vi "nanocal -- nuclear schottky fit V8.vi"() -> ()   [LabVIEW 2021] (continued)
\"τ22\" -> 0.000000000000   ,  \"τN1\" -> 0.000000000000   ,  \"τN2\" -> 0.000000000000   ,  \"σηlogτ1 \" -> 0.000000000000   ,  \"σηlogτS\" -> 0.000000000000   ,  \"σηlogτN\" -> 0.000000000000   ,  \"σlogτ1\" -> 0.000000000000   ,  \"σlogτS\" -> 0.000000000000   ,  \"σlogτN\" -> 0.000000000000   ,  \"σητ1\" -> 0.000000000000   ,  \"σητS \" -> 0.000000000000   ,  \"σητN\" -> 0.000000000000    |>   , \r\"IDS0361_210908_RAW_cal__ref_\" ->   <|    \"ζ\" -> 0.274843315726   ,  \"τ1\" -> 0.065669556126   ,  \"τS\" -> 0.043737045326   ,  \"τN\" -> 0.171424826572   ,  \"τC\" -> 0.000899266573   ,  \"κ0\" -> 0.000000000755   ,  \"mm1\" -> 0.000191414578   ,  \"mm2\" -> 0.011258128300   ,  \"mm3\" -> 0.329416954010   ,  \"T\" -> 0.168000000000   ,  \"B\" -> 12.000000000000   ,  \"θ\" -> 60.000000000000   ,  \"Reoff\" -> 0.000000000000   ,  \"Imoff\" -> 0.000000000000   ,  \"στ1\" -> 0.000077610156   ,  \"στS\" -> 0.000022738638   ,  \"στN\" -> 0.000144137782   ,  \"τ11 \" -> 0.000000000000   ,  \"τ12\" -> 0.000000000000   ,  \"τ22\" -> 0.000000000000   ,  \"τN1\" -> 0.000000000000   ,  \"τN2\" -> 0.000000000000   ,  \"σηlogτ1 \" -> 0.041134517971   ,  \"σηlogτS\" -> 0.001768570492   ,  \"σηlogτN\" -> 0.052373530031   ,  \"σlogτ1\" -> 0.001181828544   ,  \"σlogτS\" -> 0.000519894231   ,  \"σlogτN\" -> 0.000840822097   ,  \"σητ1\" -> 0.002701285537   ,  \"σητS \" -> 0.000077352048   ,  \"σητN\" -> 0.008978123302    |>   , \r\"IDS0361_210908_RAW_cal__sam_\" ->   <|    \"ζ\" -> 0.166104690940   ,  \"τ1\" -> 0.071049175548   ,  \"τS\" -> 0.068661809155   ,  \"τN\" -> 0.222482953546   ,  \"τC\" -> 0.001364223445   ,  \"κ0\" -> 0.000000000861   ,  \"mm1\" -> 0.000191495940   ,  \"mm2\" -> 0.014533832786   ,  \"mm3\" -> 0.397193343795   ,  \"T\" -> 0.168000000000   ,  \"B\" -> 12.000000000000   ,  \"θ\" -> 60.000000000000   ,  \"Reoff\" -> -34789156.626506023100   ,  \"Imoff\" -> 0.000000000000   ,  \"στ1\" -> 0.000000000000   ,  \"στS\" -> 0.000000000000   ,  \"στN\" -> 0.000000000000   ,  \"τ11 \" -> 0.000000000000   ,  \"τ12\" -> 0.000000000000   ,  \"τ22\" -> 0.000000000000   ,  \"τN1\" -> 0.000000000000   ,  \"τN2\" -> 0.000000000000   ,  \"σηlogτ1 \" -> 0.000000000000   ,  \"σηlogτS\" -> 0.000000000000   ,  \"σηlogτN\" -> 0.000000000000   ,  \"σlogτ1\" -> 0.000000000000   ,  \"σlogτS\" -> 0.000000000000   ,  \"σlogτN\" -> 0.000000000000   ,  \"σητ1\" -> 0.000000000000   ,  \"σητS \" -> 0.000000000000   ,  \"σητN\" -> 0.000000000000    |>   , \r\"IDS0362_210908_RAW_cal__ref_\" ->   <|    \"ζ\" -> 0.210826162252   ,  \"τ1\" -> 0.054763021259   ,  \"τS\" -> 0.037603010957   ,  \"τN\" -> 0.089871422671   ,  \"τC\" -> 0.000959483183   ,  \"κ0\" -> 0.000000001045   ,  \"mm1\" -> 0.000164174443   ,  \"mm2\" -> 0.012877562256   ,  \"mm3\" -> 0.197030146997   ,  \"T\" -> 0.197000000000   ,  \"B\" -> 12.000000000000   ,  \"θ\" -> 60.000000000000   ,  \"Reoff\" -> 0.000000000000   ,  \"Imoff\" -> 0.000000000000   ,  \"στ1\" -> 0.000049220168   ,  \"στS\" -> 0.000011686979   ,  \"στN\" -> 0.000056446769   ,  \"τ11 \" -> 0.000000000000   ,  \"τ12\" -> 0.000000000000   ,  \"τ22\" -> 0.000000000000   ,  \"τN1\" -> 0.000000000000   ,  \"τN2\" -> 0.000000000000   ,  \"σηlogτ1 \" -> 0.038148915938   ,  \"σηlogτS\" -> 0.001374810052   ,  \"σηlogτN\" -> 0.048522876787   ,  \"σlogτ1\" -> 0.000898784750   ,  \"σlogτS\" -> 0.000310799031   ,  \"σlogτN\" -> 0.000628083622   ,  \"σητ1\" -> 0.002089149895   ,  \"σητS \" -> 0.000051696997   ,  \"σητN\" -> 0.004360819969    |>   , \r\"IDS0362_210908_RAW_cal__sam_\" ->   <|    \"ζ\" -> 0.123741217510   ,  \"τ1\" -> 0.059103977068   ,  \"τS\" -> 0.051096152058   ,  \"τN\" -> 0.122661863704   ,  \"τC\" -> 0.001502836172   ,  \"κ0\" -> 0.000000001149   ,  \"mm1\" -> 0.000161683871   ,  \"mm2\" -> 0.014394250129   ,  \"mm3\" -> 0.241309923424   ,  \"T\" -> 0.197000000000   ,  \"B\" -> 12.000000000000   ,  \"θ\" -> 60.000000000000   ,  \"Reoff\" -> -17448795.180722892300   ,  \"Imoff\" -> 0.000000000000   ,  \"στ1\" -> 0.000000000000   ,  \"στS\" -> 0.000000000000   ,  \"στN\" -> 0.000000000000   ,  \"τ11 \" -> 0.000000000000   ,  \"τ12\" -> 0.000000000000   ,  \"τ22\" -> 0.000000000000   ,  \"τN1\" -> 0.000000000000   ,  \"τN2\" -> 0.000000000000   ,  \"σηlogτ1 \" -> 0.000000000000   ,  \"σηlogτS\" -> 0.000000000000   ,  \"σηlogτN\" -> 0.000000000000   ,  \"σlogτ1\" -> 0.000000000000   ,  \"σlogτS\" -> 0.000000000000   ,  \"σlogτN\" -> 0.000000000000   ,  \"σητ1\" -> 0.000000000000   ,  \"σητS \" -> 0.000000000000   ,  \"σητN\" -> 0.000000000000    |>   , \r\"IDS0363_210908_RAW_cal__ref_\" ->   <|    \"ζ\" -> 0.120195011159   ,  \"τ1\" -> 0.037982415348   ,  \"τS\" -> 0.029921195592   ,  \"τN\" -> 0.032714371407   ,  \"τC\" -> 0.001103711032   ,  \"κ0\" -> 0.000000001361   ,  \"mm1\" -> 0.000115022123   ,  \"mm2\" -> 0.013740329759   ,  \"mm3\" -> 0.095394824172   ,  \"T\" -> 0.250000000000   ,  \"B\" -> 12.000000000000   ,  \"θ\" -> 60.000000000000   ,  \"Reoff\" -> 0.000000000000   ,  \"Imoff\" -> 0.000000000000   ,  \"στ1\" -> 0.000012313434   ,  \"στS\" -> 0.000002128775   ,  \"στN\" -> 0.000006964176   ,  \"τ11 \" -> 0.000000000000   ,  \"τ12\" -> 0.000000000000   ,  \"τ22\" -> 0.000000000000   ,  \"τN1\" -> 0.000000000000   ,  \"τN2\" -> 0.000000000000   ,  \"σηlogτ1 \" -> 0.037050900153   ,  \"σηlogτS\" -> 0.000901906922   ,  \"σηlogτN\" -> 0.045689519095   ,  \"σlogτ1\" -> 0.000324187744   ,  \"σlogτS\" -> 0.000071146055   ,  \"σlogτN\" -> 0.000212878182   ,  \"σητ1\" -> 0.001407282679   ,  \"σητS \" -> 0.000026986133   ,  \"σητN\" -> 0.001494703897    |>   , \r\"IDS0363_210908_RAW_cal__sam_\" ->   <|    \"ζ\" -> 0.074359211271   ,  \"τ1\" -> 0.044477620306   ,  \"τS\" -> 0.040449563551   ,  \"τN\" -> 0.044745540249   ,  \"τC\" -> 0.001712765821   ,  \"κ0\" -> 0.000000001493   ,  \"mm1\" -> 0.000114327803   ,  \"mm2\" -> 0.016556677808   ,  \"mm3\" -> 0.121049525039   ,  \"T\" -> 0.250000000000   ,  \"B\" -> 12.000000000000   ,  \"θ\" -> 60.000000000000   ,  \"Reoff\" -> -10147590.361445784600   ,  \"Imoff\" -> 0.000000000000   ,  \"στ1\" -> 0.000000000000   ,  \"στS\" -> 0.000000000000   ,  \"στN\" -> 0.000000000000   ,  \"τ11 \" -> 0.000000000000   ,  \"τ12\" -> 0.000000000000   ,  \"τ22\" -> 0.000000000000   ,  \"τN1\" -> 0.000000000000   ,  \"τN2\" -> 0.000000000000   ,  \"σηlogτ1 \" -> 0.000000000000   ,  \"σηlogτS\" -> 0.000000000000   ,  \"σηlogτN\" -> 0.000000000000   ,  \"σlogτ1\" -> 0.000000000000   ,  \"σlogτS\" -> 0.000000000000   ,  \"σlogτN\" -> 0.000000000000   ,  \"σητ1\" -> 0.000000000000   ,  \"σητS \" -> 0.000000000000   ,  \"σητN\" -> 0.000000000000    |>   , \r\"IDS0364_210908_RAW_cal__ref_\" ->   <|    \"ζ\" -> 0.081935948170   ,  \"τ1\" -> 0.032287614632   ,  \"τS\" -> 0.026949270434   ,  \"τN\" -> 0.016861876648   ,  \"τC\" -> 0.001338410345   ,  \"κ0\" -> 0.000000001744   ,  \"mm1\" -> 0.000097212898   ,  \"mm2\" -> 0.014855671361   ,  \"mm3\" -> 0.066073995677   ,  \"T\" -> 0.307000000000   ,  \"B\" -> 12.000000000000   ,  \"θ\" -> 60.000000000000   ,  \"Reoff\" -> 0.000000000000   ,  \"Imoff\" -> 0.000000000000   ,  \"στ1\" -> 0.000017118957   ,  \"στS\" -> 0.000002077535   ,  \"στN\" -> 0.000005632909   ,  \"τ11 \" -> 0.000000000000   ,  \"τ12\" -> 0.000000000000   ,  \"τ22\" -> 0.000000000000   ,  \"τN1\" -> 0.000000000000   ,  \"τN2\" -> 0.000000000000   ,  \"σηlogτ1 \" -> 0.036879495168   ,  \"σηlogτS\" -> 0.000607281388   ,  \"σηlogτN\" -> 0.044616936261   ,  \"σlogτ1\" -> 0.000530201983   ,  \"σlogτS\" -> 0.000077090575   ,  \"σlogτN\" -> 0.000334061782   ,  \"σητ1\" -> 0.001190750928   ,  \"σητS \" -> 0.000016365790   ,  \"σητN\" -> 0.000752325276    |>   , \r\"IDS0364_210908_RAW_cal__sam_\" ->   <|    \"ζ\" -> 0.051560123380   ,  \"τ1\" -> 0.037167172913   ,  \"τS\" -> 0.035875072163   ,  \"τN\" -> 0.021782945969   ,  \"τC\" -> 0.002191662682   ,  \"κ0\" -> 0.000000001902   ,  \"mm1\" -> 0.000101812126   ,  \"mm2\" -> 0.018093196790   ,  \"mm3\" -> 0.081794699340   ,  \"T\" -> 0.307000000000   ,  \"B\" -> 12.000000000000   ,  \"θ\" -> 60.000000000000   ,  \"Reoff\" -> -5584337.349397592250   ,  \"Imoff\" -> 0.000000000000   ,  \"στ1\" -> 0.000000000000   ,  \"στS\" -> 0.000000000000   ,  \"στN\" -> 0.000000000000   ,  \"τ11 \" -> 0.000000000000   ,  \"τ12\" -> 0.000000000000   ,  \"τ22\" -> 0.000000000000   ,  \"τN1\" -> 0.000000000000   ,  \"τN2\" -> 0.000000000000   ,  \"σηlogτ1 \" -> 0.000000000000   ,  \"σηlogτS\" -> 0.000000000000   ,  \"σηlogτN\" -> 0.000000000000   ,  \"σlogτ1\" -> 0.000000000000   ,  \"σlogτS\" -> 0.000000000000   ,  \"σlogτN\" -> 0.000000000000   ,  \"σητ1\" -> 0.000000000000   ,  \"σητS \" -> 0.000000000000   ,  \"σητN\" -> 0.000000000000    |>   , \r\"IDS0365_210908_RAW_cal__ref_\" ->   <|    \"ζ\" -> 0.060609447021   ,  \"τ1\" -> 0.026924433713   ,  \"τS\" -> 0.025092686079   ,  \"τN\" -> 0.009588284117   ,  \"τC\" -> 0.001648006453   ,  \"κ0\" -> 0.000000002119   ,  \"mm1\" -> 0.000088958851   ,  \"mm2\" -> 0.015130564959   ,  \"mm3\" -> 0.050135880977   ,  \"T\" -> 0.360000000000   ,  \"B\" -> 12.000000000000   ,  \"θ\" -> 60.000000000000   ,  \"Reoff\" -> 0.000000000000   ,  \"Imoff\" -> 0.000000000000   ,  \"στ1\" -> 0.000013873165   ,  \"στS\" -> 0.000001316641   ,  \"στN\" -> 0.000002948025   ,  \"τ11 \" -> 0.000000000000   ,  \"τ12\" -> 0.000000000000   ,  \"τ22\" -> 0.000000000000   ,  \"τN1\" -> 0.000000000000   ,  \"τN2\" -> 0.000000000000   ,  \"σηlogτ1 \" -> 0.038447991520   ,  \"σηlogτS\" -> 0.000466260948   ,  \"σηlogτN\" -> 0.044499975786   ,  \"σlogτ1\" -> 0.000515263014   ,  \"σlogτS\" -> 0.000052471110   ,  \"σlogτN\" -> 0.000307461145   ,  \"σητ1\" -> 0.001035190399   ,  \"σητS \" -> 0.000011699740   ,  \"σητN\" -> 0.000426678411    |>   , \r\"IDS0365_210908_RAW_cal__sam_\" ->   <|    \"ζ\" -> 0.037527154631   ,  \"τ1\" -> 0.031791574880   ,  \"τS\" -> 0.032568278603   ,  \"τN\" -> 0.012463984296   ,  \"τC\" -> 0.002682405917   ,  \"κ0\" -> 0.000000002306   ,  \"mm1\" -> 0.000090102201   ,  \"mm2\" -> 0.018466994147   ,  \"mm3\" -> 0.062639080041   ,  \"T\" -> 0.360000000000   ,  \"B\" -> 12.000000000000   ,  \"θ\" -> 60.000000000000   ,  \"Reoff\" -> -2846385.542168676850   ,  \"Imoff\" -> 0.000000000000   ,  \"στ1\" -> 0.000000000000   ,  \"στS\" -> 0.000000000000   ,  \"στN\" -> 0.000000000000   ,  \"τ11 \" -> 0.000000000000   ,  \"τ12\" -> 0.000000000000   ,  \"τ22\" -> 0.000000000000   ,  \"τN1\" -> 0.000000000000   ,  \"τN2\" -> 0.000000000000   ,  \"σηlogτ1 \" -> 0.000000000000   ,  \"σηlogτS\" -> 0.000000000000   ,  \"σηlogτN\" -> 0.000000000000   ,  \"σlogτ1\" -> 0.000000000000   ,  \"σlogτS\" -> 0.000000000000   ,  \"σlogτN\" -> 0.000000000000   ,  \"σητ1\" -> 0.000000000000   ,  \"σητS \" -> 0.000000000000   ,  \"σητN\" -> 0.000000000000    |>   , \r\"IDS0366_210908_RAW_cal__ref_\" ->   <|    \"ζ\" -> 0.044599134979   ,  \"τ1\" -> 0.022455429279   ,  \"τS\" -> 0.023337915843   ,  \"τN\" -> 0.005128755710   ,  \"τC\" -> 0.001792889841   ,  \"κ0\" -> 0.000000002649   ,  \"mm1\" -> 0.000071495516   ,  \"mm2\" -> 0.015101682830   ,  \"mm3\" -> 0.038811401254   ,  \"T\" -> 0.430000000000   ,  \"B\" -> 12.000000000000   ,  \"θ\" -> 60.000000000000   ,  \"Reoff\" -> 0.000000000000   ,  \"Imoff\" -> 0.000000000000   ,  \"στ1\" -> 0.000015607545   ,  \"στS\" -> 0.000001063228   ,  \"στN\" -> 0.000002022209   ,  \"τ11 \" -> 0.000000000000   ,  \"τ12\" -> 0.000000000000   ,  \"τ22\" -> 0.000000000000   ,  \"τN1\" -> 0.000000000000   ,  \"τN2\" -> 0.000000000000   ,  \"σηlogτ1 \" -> 0.040328561350   ,  \"σηlogτS\" -> 0.000330725156   ,  \"σηlogτN\" -> 0.044548205014   ,  \"σlogτ1\" -> 0.000695045482   ,  \"σlogτS\" -> 0.000045557962   ,  \"σlogτN\" -> 0.000394288447   ,  \"σητ1\" -> 0.000905595157   ,  \"σητS \" -> 0.000007718436   ,  \"σητN\" -> 0.000228476861    |>   , \r\"IDS0366_210908_RAW_cal__sam_\" ->   <|    \"ζ\" -> 0.029143715364   ,  \"τ1\" -> 0.026198855926   ,  \"τS\" -> 0.029745373312   ,  \"τN\" -> 0.006649011545   ,  \"τC\" -> 0.003090491846   ,  \"κ0\" -> 0.000000002869   ,  \"mm1\" -> 0.000079676072   ,  \"mm2\" -> 0.018163106475   ,  \"mm3\" -> 0.048501617675   ,  \"T\" -> 0.430000000000   ,  \"B\" -> 12.000000000000   ,  \"θ\" -> 60.000000000000   ,  \"Reoff\" -> -2237951.807228915390   ,  \"Imoff\" -> 0.000000000000   ,  \"στ1\" -> 0.000000000000   ,  \"στS\" -> 0.000000000000   ,  \"στN\" -> 0.000000000000   ,  \"τ11 \" -> 0.000000000000   ,  \"τ12\" -> 0.000000000000   ,  \"τ22\" -> 0.000000000000   ,  \"τN1\" -> 0.000000000000   ,  \"τN2\" -> 0.000000000000   ,  \"σηlogτ1 \" -> 0.000000000000   ,  \"σηlogτS\" -> 0.000000000000   ,  \"σηlogτN\" -> 0.000000000000   ,  \"σlogτ1\" -> 0.000000000000   ,  \"σlogτS\" -> 0.000000000000   ,  \"σlogτN\" -> 0.000000000000   ,  \"σητ1\" -> 0.000000000000   ,  \"σητS \" -> 0.000000000000   ,  \"σητN\" -> 0.000000000000    |>   , \r\"IDS0367_210908_RAW_cal__ref_\" ->   <|    \"ζ\" -> 0.034740009221   ,  \"τ1\" -> 0.017028751834   ,  \"τS\" -> 0.022162435410   ,  \"τN\" -> 0.002809238258   ,  \"τC\" -> 0.001913219314   ,  \"κ0\" -> 0.000000003308   ,  \"mm1\" -> 0.000059427665   ,  \"mm2\" -> 0.013533798262   ,  \"mm3\" -> 0.031187935063   ,  \"T\" -> 0.530000000000   ,  \"B\" -> 12.000000000000   ,  \"θ\" -> 60.000000000000   ,  \"Reoff\" -> 0.000000000000   ,  \"Imoff\" -> 0.000000000000   ,  \"στ1\" -> 0.000027033003   ,  \"στS\" -> 0.000001554115   ,  \"στN\" -> 0.000002352999   ,  \"τ11 \" -> 0.000000000000   ,  \"τ12\" -> 0.000000000000   ,  \"τ22\" -> 0.000000000000   ,  \"τN1\" -> 0.000000000000   ,  \"τN2\" -> 0.000000000000   ,  \"σηlogτ1 \" -> 0.045416924257   ,  \"σηlogτS\" -> 0.000278228215   ,  \"σηlogτN\" -> 0.045395504019   ,  \"σlogτ1\" -> 0.001587491763   ,  \"σlogτS\" -> 0.000070123814   ,  \"σlogτN\" -> 0.000837593181   ,  \"σητ1\" -> 0.000773393532   ,  \"σητS \" -> 0.000006166215   ,  \"σητN\" -> 0.000127526787    |>   , \r\"IDS0367_210908_RAW_cal__sam_\" ->   <|    \"ζ\" -> 0.024637271207   ,  \"τ1\" -> 0.025634847148   ,  \"τS\" -> 0.027302474030   ,  \"τN\" -> 0.003538185279   ,  \"τC\" -> 0.003933377133   ,  \"κ0\" -> 0.000000003566   ,  \"mm1\" -> 0.000083131278   ,  \"mm2\" -> 0.019726981228   ,  \"mm3\" -> 0.041358600771   ,  \"T\" -> 0.530000000000   ,  \"B\" -> 12.000000000000   ,  \"θ\" -> 60.000000000000   ,  \"Reoff\" -> -1629518.072289161380   ,  \"Imoff\" -> 0.000000000000   ,  \"στ1\" -> 0.000000000000   ,  \"στS\" -> 0.000000000000   ,  \"στN\" -> 0.000000000000   ,  \"τ11 \" -> 0.000000000000   ,  \"τ12\" -> 0.000000000000   ,  \"τ22\" -> 0.000000000000   ,  \"τN1\" -> 0.000000000000   ,  \"τN2\" -> 0.000000000000   ,  \"σηlogτ1 \" -> 0.000000000000   ,  \"σηlogτS\" -> 0.000000000000   ,  \"σηlogτN\" -> 0.000000000000   ,  \"σlogτ1\" -> 0.000000000000   ,  \"σlogτS\" -> 0.000000000000   ,  \"σlogτN\" -> 0.000000000000   ,  \"σητ1\" -> 0.000000000000   ,  \"σητS \" -> 0.000000000000   ,  \"σητN\" -> 0.000000000000    |>   , \r\"IDS0368_210908_RAW_cal__ref_\" ->   <|    \"ζ\" -> 0.027231595728   ,  \"τ1\" -> 0.015050030834   ,  \"τS\" -> 0.020840826339   ,  \"τN\" -> 0.001677171050   ,  \"τC\" -> 0.002801092038   ,  \"κ0\" -> 0.000000003924   ,  \"mm1\" -> 0.000065840915   ,  \"mm2\" -> 0.013031059806   ,  \"mm3\" -> 0.027885420541   ,  \"T\" -> 0.630000000000   ,  \"B\" -> 12.000000000000   ,  \"θ\" -> 60.000000000000   ,  \"Reoff\" -> 0.000000000000   ,  \"Imoff\" -> 0.000000000000   ,  \"στ1\" -> 0.000025618780   ,  \"στS\" -> 0.000001064388   ,  \"στN\" -> 0.000001464284   ,  \"τ11 \" -> 0.000000000000   ,  \"τ12\" -> 0.000000000000   ,  \"τ22\" -> 0.000000000000   ,  \"τN1\" -> 0.000000000000   ,  \"τN2\" -> 0.000000000000   ,  \"σηlogτ1 \" -> 0.047954951123   ,  \"σηlogτS\" -> 0.000209073519   ,  \"σηlogτN\" -> 0.045696441574   ,  \"σlogτ1\" -> 0.001702241050   ,  \"σlogτS\" -> 0.000051072269   ,  \"σlogτN\" -> 0.000873068059   ,  \"σητ1\" -> 0.000721723493   ,  \"σητS \" -> 0.000004357265   ,  \"σητN\" -> 0.000076640749    |>   , \r\"IDS0368_210908_RAW_cal__sam_\" ->   <|    \"ζ\" -> 0.021420270760   ,  \"τ1\" -> 0.018208454683   ,  \"τS\" -> 0.024985612374   ,  \"τN\" -> 0.002144760910   ,  \"τC\" -> 0.004931614434   ,  \"κ0\" -> 0.000000004254   ,  \"mm1\" -> 0.000086915042   ,  \"mm2\" -> 0.015826314138   ,  \"mm3\" -> 0.034938353162   ,  \"T\" -> 0.630000000000   ,  \"B\" -> 12.000000000000   ,  \"θ\" -> 60.000000000000   ,  \"Reoff\" -> -1204819.277108438310   ,  \"Imoff\" -> 0.000000000000   ,  \"στ1\" -> 0.000000000000   ,  \"στS\" -> 0.000000000000   ,  \"στN\" -> 0.000000000000   ,  \"τ11 \" -> 0.000000000000   ,  \"τ12\" -> 0.000000000000   ,  \"τ22\" -> 0.000000000000   ,  \"τN1\" -> 0.000000000000   ,  \"τN2\" -> 0.000000000000   ,  \"σηlogτ1 \" -> 0.000000000000   ,  \"σηlogτS\" -> 0.000000000000   ,  \"σηlogτN\" -> 0.000000000000   ,  \"σlogτ1\" -> 0.000000000000   ,  \"σlogτS\" -> 0.000000000000   ,  \"σlogτN\" -> 0.000000000000   ,  \"σητ1\" -> 0.000000000000   ,  \"σητS \" -> 0.000000000000   ,  \"σητN\" -> 0.000000000000    |>   , \r\"IDS0369_210908_RAW_cal__ref_\" ->   <|    \"ζ\" -> 0.020332946442   ,  \"τ1\" -> 0.011808248331   ,  \"τS\" -> 0.019124131146   ,  \"τN\" -> 0.000708402175   ,  \"τC\" -> 0.003056309257   ,  \"κ0\" -> 0.000000005441   ,  \"mm1\" -> 0.000052779905   ,  \"mm2\" -> 0.011105332134   ,  \"mm3\" -> 0.023942232708   ,  \"T\" -> 0.830000000000   ,  \"B\" -> 12.000000000000   ,  \"θ\" -> 60.000000000000   ,  \"Reoff\" -> 0.000000000000   ,  \"Imoff\" -> 0.000000000000   ,  \"στ1\" -> 0.000047094116   ,  \"στS\" -> 0.000001159219   ,  \"στN\" -> 0.000001405585   ,  \"τ11 \" -> 0.000000000000   ,  \"τ12\" -> 0.000000000000   ,  \"τ22\" -> 0.000000000000   ,  \"τN1\" -> 0.000000000000   ,  \"τN2\" -> 0.000000000000   ,  \"σηlogτ1 \" -> 0.053002916420   ,  \"σηlogτS\" -> 0.000126082533   ,  \"σηlogτN\" -> 0.046399219380   ,  \"σlogτ1\" -> 0.003988238919   ,  \"σlogτS\" -> 0.000060615502   ,  \"σlogτN\" -> 0.001984162345   ,  \"σητ1\" -> 0.000625871599   ,  \"σητS \" -> 0.000002411219   ,  \"σητN\" -> 0.000032869308    |>   , \r\"IDS0369_210908_RAW_cal__sam_\" ->   <|    \"ζ\" -> 0.014606512986   ,  \"τ1\" -> 0.019756664879   ,  \"τS\" -> 0.022303249954   ,  \"τN\" -> 0.001023812506   ,  \"τC\" -> 0.005490022400   ,  \"κ0\" -> 0.000000005866   ,  \"mm1\" -> 0.000063747249   ,  \"mm2\" -> 0.017921258799   ,  \"mm3\" -> 0.030929470731   ,  \"T\" -> 0.830000000000   ,  \"B\" -> 12.000000000000   ,  \"θ\" -> 60.000000000000   ,  \"Reoff\" -> -481927.710843376814   ,  \"Imoff\" -> 0.000000000000   ,  \"στ1\" -> 0.000000000000   ,  \"στS\" -> 0.000000000000   ,  \"στN\" -> 0.000000000000   ,  \"τ11 \" -> 0.000000000000   ,  \"τ12\" -> 0.000000000000   ,  \"τ22\" -> 0.000000000000   ,  \"τN1\" -> 0.000000000000   ,  \"τN2\" -> 0.000000000000   ,  \"σηlogτ1 \" -> 0.000000000000   ,  \"σηlogτS\" -> 0.000000000000   ,  \"σηlogτN\" -> 0.000000000000   ,  \"σlogτ1\" -> 0.000000000000   ,  \"σlogτS\" -> 0.000000000000   ,  \"σlogτN\" -> 0.000000000000   ,  \"σητ1\" -> 0.000000000000   ,  \"σητS \" -> 0.000000000000   ,  \"σητN\" -> 0.000000000000    |>   , \r\"IDS0370_210908_RAW_cal__ref_\" ->   <|    \"ζ\" -> 0.016443978585   ,  \"τ1\" -> 0.012644854996   ,  \"τS\" -> 0.017634511441   ,  \"τN\" -> 0.000316227766   ,  \"τC\" -> 0.002708386911   ,  \"κ0\" -> 0.000000007589   ,  \"mm1\" -> 0.000038134808   ,  \"mm2\" -> 0.012179834504   ,  \"mm3\" -> 0.021381193373   ,  \"T\" -> 1.130000000000   ,  \"B\" -> 12.000000000000   ,  \"θ\" -> 60.000000000000   ,  \"Reoff\" -> 0.000000000000   ,  \"Imoff\" -> 0.000000000000   ,  \"στ1\" -> 0.000121213865   ,  \"στS\" -> 0.000001160231   ,  \"στN\" -> 0.000001536991   ,  \"τ11 \" -> 0.000000000000   ,  \"τ12\" -> 0.000000000000   ,  \"τ22\" -> 0.000000000000   ,  \"τN1\" -> 0.000000000000   ,  \"τN2\" -> 0.000000000000   ,  \"σηlogτ1 \" -> 0.048314482275   ,  \"σηlogτS\" -> 0.000048505756   ,  \"σηlogτN\" -> 0.045503358655   ,  \"σlogτ1\" -> 0.009586022574   ,  \"σlogτS\" -> 0.000065793194   ,  \"σlogτN\" -> 0.004860390947   ,  \"σητ1\" -> 0.000610929623   ,  \"σητS \" -> 0.000000855375   ,  \"σητN\" -> 0.000014389425    |>   , \r\"IDS0370_210908_RAW_cal__sam_\" ->   <|    \"ζ\" -> 0.013427569249   ,  \"τ1\" -> 0.019934074843   ,  \"τS\" -> 0.019524726442   ,  \"τN\" -> 0.000513623253   ,  \"τC\" -> 0.005657316251   ,  \"κ0\" -> 0.000000008143   ,  \"mm1\" -> 0.000058424467   ,  \"mm2\" -> 0.018528796956   ,  \"mm3\" -> 0.027311585694   ,  \"T\" -> 1.130000000000   ,  \"B\" -> 12.000000000000   ,  \"θ\" -> 60.000000000000   ,  \"Reoff\" -> -481927.710843376814   ,  \"Imoff\" -> 0.000000000000   ,  \"στ1\" -> 0.000000000000   ,  \"στS\" -> 0.000000000000   ,  \"στN\" -> 0.000000000000   ,  \"τ11 \" -> 0.000000000000   ,  \"τ12\" -> 0.000000000000   ,  \"τ22\" -> 0.000000000000   ,  \"τN1\" -> 0.000000000000   ,  \"τN2\" -> 0.000000000000   ,  \"σηlogτ1 \" -> 0.000000000000   ,  \"σηlogτS\" -> 0.000000000000   ,  \"σηlogτN\" -> 0.000000000000   ,  \"σlogτ1\" -> 0.000000000000   ,  \"σlogτS\" -> 0.000000000000   ,  \"σlogτN\" -> 0.000000000000   ,  \"σητ1\" -> 0.000000000000   ,  \"σητS \" -> 0.000000000000   ,  \"σητN\" -> 0.000000000000    |>   , \r\"IDS0371_210908_RAW_cal__ref_\" ->   <|    \"ζ\" -> 0.020664849580   ,  \"τ1\" -> 0.018108723176   ,  \"τS\" -> 0.010299896170   ,  \"τN\" -> 0.000079818017   ,  \"τC\" -> 0.006259144045   ,  \"κ0\" -> 0.000000013130   ,  \"mm1\" -> 0.000079811267   ,  \"mm2\" -> 0.016056535433   ,  \"mm3\" -> 0.018825729941   ,  \"T\" -> 1.900000000000   ,  \"B\" -> 12.000000000000   ,  \"θ\" -> 60.000000000000   ,  \"Reoff\" -> 0.000000000000   ,  \"Imoff\" -> 0.000000000000   ,  \"στ1\" -> 0.000000000000   ,  \"στS\" -> 0.000000000000   ,  \"στN\" -> 0.000000000000   ,  \"τ11 \" -> 0.000000000000   ,  \"τ12\" -> 0.000000000000   ,  \"τ22\" -> 0.000000000000   ,  \"τN1\" -> 0.000000000000   ,  \"τN2\" -> 0.000000000000   ,  \"σηlogτ1 \" -> 0.000000000000   ,  \"σηlogτS\" -> 0.000000000000   ,  \"σηlogτN\" -> 0.000000000000   ,  \"σlogτ1\" -> 0.000000000000   ,  \"σlogτS\" -> 0.000000000000   ,  \"σlogτN\" -> 0.000000000000   ,  \"σητ1\" -> 0.000000000000   ,  \"σητS \" -> 0.000000000000   ,  \"σητN\" -> 0.000000000000    |>   , \r\"IDS0371_210908_RAW_cal__sam_\" ->   <|    \"ζ\" -> 0.009645933094   ,  \"τ1\" -> 0.020976887035   ,  \"τS\" -> 0.013140254521   ,  \"τN\" -> 0.000215522697   ,  \"τC\" -> 0.007317042194   ,  \"κ0\" -> 0.000000013897   ,  \"mm1\" -> 0.000045154509   ,  \"mm2\" -> 0.018728618799   ,  \"mm3\" -> 0.023004762073   ,  \"T\" -> 1.900000000000   ,  \"B\" -> 12.000000000000   ,  \"θ\" -> 60.000000000000   ,  \"Reoff\" -> -120481.927710846066   ,  \"Imoff\" -> 0.000000000000   ,  \"στ1\" -> 0.000000000000   ,  \"στS\" -> 0.000000000000   ,  \"στN\" -> 0.000000000000   ,  \"τ11 \" -> 0.000000000000   ,  \"τ12\" -> 0.000000000000   ,  \"τ22\" -> 0.000000000000   ,  \"τN1\" -> 0.000000000000   ,  \"τN2\" -> 0.000000000000   ,  \"σηlogτ1 \" -> 0.000000000000   ,  \"σηlogτS\" -> 0.000000000000   ,  \"σηlogτN\" -> 0.000000000000   ,  \"σlogτ1\" -> 0.000000000000   ,  \"σlogτS\" -> 0.000000000000   ,  \"σlogτN\" -> 0.000000000000   ,  \"σητ1\" -> 0.000000000000   ,  \"σητS \" -> 0.000000000000   ,  \"σητN\" -> 0.000000000000    |>   , \r\"IDS0372_210908_RAW_cal__ref_\" ->   <|    \"ζ\" -> 0.021592146431   ,  \"τ1\" -> 0.018093446545   ,  \"τS\" -> 0.007071841556   ,  \"τN\" -> 0.000029085223   ,  \"τC\" -> 0.005341206531   ,  \"κ0\" -> 0.000000023517   ,  \"mm1\" -> 0.000065243548   ,  \"mm2\" -> 0.012435446609   ,  \"mm3\" -> 0.018188213949   ,  \"T\" -> 3.110000000000   ,  \"B\" -> 12.000000000000   ,  \"θ\" -> 60.000000000000   ,  \"Reoff\" -> 0.000000000000   ,  \"Imoff\" -> 0.000000000000   ,  \"στ1\" -> 0.000000000000   ,  \"στS\" -> 0.000000000000   ,  \"στN\" -> 0.000000000000   ,  \"τ11 \" -> 0.000000000000   ,  \"τ12\" -> 0.000000000000   ,  \"τ22\" -> 0.000000000000   ,  \"τN1\" -> 0.000000000000   ,  \"τN2\" -> 0.000000000000   ,  \"σηlogτ1 \" -> 0.000000000000   ,  \"σηlogτS\" -> 0.000000000000   ,  \"σηlogτN\" -> 0.000000000000   ,  \"σlogτ1\" -> 0.000000000000   ,  \"σlogτS\" -> 0.000000000000   ,  \"σlogτN\" -> 0.000000000000   ,  \"σητ1\" -> 0.000000000000   ,  \"σητS \" -> 0.000000000000   ,  \"σητN\" -> 0.000000000000    |>   , \r\"IDS0372_210908_RAW_cal__sam_\" ->   <|    \"ζ\" -> 0.010006554735   ,  \"τ1\" -> 0.021193289022   ,  \"τS\" -> 0.010059776467   ,  \"τN\" -> 0.000092737128   ,  \"τC\" -> 0.005619947239   ,  \"κ0\" -> 0.000000024358   ,  \"mm1\" -> 0.000035931477   ,  \"mm2\" -> 0.015490366222   ,  \"mm3\" -> 0.021541043840   ,  \"T\" -> 3.110000000000   ,  \"B\" -> 12.000000000000   ,  \"θ\" -> 60.000000000000   ,  \"Reoff\" -> -120481.927710846066   ,  \"Imoff\" -> 0.000000000000   ,  \"στ1\" -> 0.000000000000   ,  \"στS\" -> 0.000000000000   ,  \"στN\" -> 0.000000000000   ,  \"τ11 \" -> 0.000000000000   ,  \"τ12\" -> 0.000000000000   ,  \"τ22\" -> 0.000000000000   ,  \"τN1\" -> 0.000000000000   ,  \"τN2\" -> 0.000000000000   ,  \"σηlogτ1 \" -> 0.000000000000   ,  \"σηlogτS\" -> 0.000000000000   ,  \"σηlogτN\" -> 0.000000000000   ,  \"σlogτ1\" -> 0.000000000000   ,  \"σlogτS\" -> 0.000000000000   ,  \"σlogτN\" -> 0.000000000000   ,  \"σητ1\" -> 0.000000000000   ,  \"σητS \" -> 0.000000000000   ,  \"σητN\" -> 0.000000000000    |>   , \r\"IDS0373_210908_RAW_cal__ref_\" ->   <|    \"ζ\" -> 0.028148688120   ,  \"τ1\" -> 0.012706961955   ,  \"τS\" -> 0.003881518121   ,  \"τN\" -> 0.000007160132   ,  \"τC\" -> 0.004346615253   ,  \"κ0\" -> 0.000000058313   ,  \"mm1\" -> 0.000057355729   ,  \"mm2\" -> 0.008266435527   ,  \"mm3\" -> 0.012727925396   ,  \"T\" -> 5.750000000000   ,  \"B\" -> 12.000000000000   ,  \"θ\" -> 60.000000000000   ,  \"Reoff\" -> 0.000000000000   ,  \"Imoff\" -> 0.000000000000   ,  \"στ1\" -> 0.000000000000   ,  \"στS\" -> 0.000000000000   ,  \"στN\" -> 0.000000000000   ,  \"τ11 \" -> 0.000000000000   ,  \"τ12\" -> 0.000000000000   ,  \"τ22\" -> 0.000000000000   ,  \"τN1\" -> 0.000000000000   ,  \"τN2\" -> 0.000000000000   ,  \"σηlogτ1 \" -> 0.000000000000   ,  \"σηlogτS\" -> 0.000000000000   ,  \"σηlogτN\" -> 0.000000000000   ,  \"σlogτ1\" -> 0.000000000000   ,  \"σlogτS\" -> 0.000000000000   ,  \"σlogτN\" -> 0.000000000000   ,  \"σητ1\" -> 0.000000000000   ,  \"σητS \" -> 0.000000000000   ,  \"σητN\" -> 0.000000000000    |>   , \r\"IDS0373_210908_RAW_cal__sam_\" ->   <|    \"ζ\" -> 0.009383547393   ,  \"τ1\" -> 0.021616814113   ,  \"τS\" -> 0.006389723126   ,  \"τN\" -> 0.000031102862   ,  \"τC\" -> 0.004593168461   ,  \"κ0\" -> 0.000000059183   ,  \"mm1\" -> 0.000024995592   ,  \"mm2\" -> 0.010985466166   ,  \"mm3\" -> 0.021680596929   ,  \"T\" -> 5.750000000000   ,  \"B\" -> 12.000000000000   ,  \"θ\" -> 60.000000000000   ,  \"Reoff\" -> -40000.000000000000   ,  \"Imoff\" -> 0.000000000000   ,  \"στ1\" -> 0.000000000000   ,  \"στS\" -> 0.000000000000   ,  \"στN\" -> 0.000000000000   ,  \"τ11 \" -> 0.000000000000   ,  \"τ12\" -> 0.000000000000   ,  \"τ22\" -> 0.000000000000   ,  \"τN1\" -> 0.000000000000   ,  \"τN2\" -> 0.000000000000   ,  \"σηlogτ1 \" -> 0.000000000000   ,  \"σηlogτS\" -> 0.000000000000   ,  \"σηlogτN\" -> 0.000000000000   ,  \"σlogτ1\" -> 0.000000000000   ,  \"σlogτS\" -> 0.000000000000   ,  \"σlogτN\" -> 0.000000000000   ,  \"σητ1\" -> 0.000000000000   ,  \"σητS \" -> 0.000000000000   ,  \"σητN\" -> 0.000000000000    |>   , \r\"IDS0377_210909_RAW_cal__ref_\" ->   <|    \"ζ\" -> 0.246550605323   ,  \"τ1\" -> 0.063098036224   ,  \"τS\" -> 0.035636106163   ,  \"τN\" -> 0.021974547329   ,  \"τC\" -> 0.000821092988   ,  \"κ0\" -> 0.000000001041   ,  \"mm1\" -> 0.000160015882   ,  \"mm2\" -> 0.025949965723   ,  \"mm3\" -> 0.109623742590   ,  \"T\" -> 0.197000000000   ,  \"B\" -> 8.000000000000   ,  \"θ\" -> 0.000000000000   ,  \"Reoff\" -> -36382320.441988945000   ,  \"Imoff\" -> 0.000000000000   ,  \"στ1\" -> 0.000062922538   ,  \"στS\" -> 0.000014967815   ,  \"στN\" -> 0.000031670740   ,  \"τ11 \" -> 0.000000000000   ,  \"τ12\" -> 0.000000000000   ,  \"τ22\" -> 0.000000000000   ,  \"τN1\" -> 0.000000000000   ,  \"τN2\" -> 0.000000000000   ,  \"σηlogτ1 \" -> 0.000000000000   ,  \"σηlogτS\" -> 0.000000000000   ,  \"σηlogτN\" -> 0.000000000000   ,  \"σlogτ1\" -> 0.000000000000   ,  \"σlogτS\" -> 0.000000000000   ,  \"σlogτN\" -> 0.000000000000   ,  \"σητ1\" -> 0.000000000000   ,  \"σητS \" -> 0.000000000000   ,  \"σητN\" -> 0.000000000000    |>   , \r\"IDS0377_210909_RAW_cal__sam_\" ->   <|    \"ζ\" -> 0.135798490691   ,  \"τ1\" -> 0.079257563336   ,  \"τS\" -> 0.046440970443   ,  \"τN\" -> 0.031537801980   ,  \"τC\" -> 0.001434159670   ,  \"κ0\" -> 0.000000001166   ,  \"mm1\" -> 0.000167444282   ,  \"mm2\" -> 0.031002991367   ,  \"mm3\" -> 0.138089459380   ,  \"T\" -> 0.197000000000   ,  \"B\" -> 8.000000000000   ,  \"θ\" -> 0.000000000000   ,  \"Reoff\" -> -18665662.650602411500   ,  \"Imoff\" -> 0.000000000000   ,  \"στ1\" -> 0.000000000000   ,  \"στS\" -> 0.000000000000   ,  \"στN\" -> 0.000000000000   ,  \"τ11 \" -> 0.000000000000   ,  \"τ12\" -> 0.000000000000   ,  \"τ22\" -> 0.000000000000   ,  \"τN1\" -> 0.000000000000   ,  \"τN2\" -> 0.000000000000   ,  \"σηlogτ1 \" -> 0.000000000000   ,  \"σηlogτS\" -> 0.000000000000   ,  \"σηlogτN\" -> 0.000000000000   ,  \"σlogτ1\" -> 0.000000000000   ,  \"σlogτS\" -> 0.000000000000   ,  \"σlogτN\" -> 0.000000000000   ,  \"σητ1\" -> 0.000000000000   ,  \"σητS \" -> 0.000000000000   ,  \"σητN\" -> 0.000000000000    |>   , \r\"IDS0378_210909_RAW_cal__ref_\" ->   <|    \"ζ\" -> 0.463349829387   ,  \"τ1\" -> 0.074237051581   ,  \"τS\" -> 0.056120726288   ,  \"τN\" -> 0.098410853279   ,  \"τC\" -> 0.000795788528   ,  \"κ0\" -> 0.000000000406   ,  \"mm1\" -> 0.000250303134   ,  \"mm2\" -> 0.022004830152   ,  \"mm3\" -> 0.278911467417   ,  \"T\" -> 0.122000000000   ,  \"B\" -> 8.000000000000   ,  \"θ\" -> 0.000000000000   ,  \"Reoff\" -> -133680722.891566262000   ,  \"Imoff\" -> 0.000000000000   ,  \"στ1\" -> 0.000032928627   ,  \"στS\" -> 0.000022172362   ,  \"στN\" -> 0.000014961504   ,  \"τ11 \" -> 0.000000000000   ,  \"τ12\" -> 0.000000000000   ,  \"τ22\" -> 0.000000000000   ,  \"τN1\" -> 0.000000000000   ,  \"τN2\" -> 0.000000000000   ,  \"σηlogτ1 \" -> 0.000000000000   ,  \"σηlogτS\" -> 0.000000000000   ,  \"σηlogτN\" -> 0.000000000000   ,  \"σlogτ1\" -> 0.000000000000   ,  \"σlogτS\" -> 0.000000000000   ,  \"σlogτN\" -> 0.000000000000   ,  \"σητ1\" -> 0.000000000000   ,  \"σητS \" -> 0.000000000000   ,  \"σητN\" -> 0.000000000000    |>   , \r\"IDS0378_210909_RAW_cal__sam_\" ->   <|    \"ζ\" -> 0.261650469875   ,  \"τ1\" -> 0.181870145043   ,  \"τS\" -> 0.168113301561   ,  \"τN\" -> 0.186965229666   ,  \"τC\" -> 0.001543998203   ,  \"κ0\" -> 0.000000000530   ,  \"mm1\" -> 0.000318362571   ,  \"mm2\" -> 0.069029342513   ,  \"mm3\" -> 0.562051433928   ,  \"T\" -> 0.122000000000   ,  \"B\" -> 8.000000000000   ,  \"θ\" -> 0.000000000000   ,  \"Reoff\" -> -63674698.795180723100   ,  \"Imoff\" -> 0.000000000000   ,  \"στ1\" -> 0.000000000000   ,  \"στS\" -> 0.000000000000   ,  \"στN\" -> 0.000000000000   ,  \"τ11 \" -> 0.000000000000   ,  \"τ12\" -> 0.000000000000   ,  \"τ22\" -> 0.000000000000   ,  \"τN1\" -> 0.000000000000   ,  \"τN2\" -> 0.000000000000   ,  \"σηlogτ1 \" -> 0.000000000000   ,  \"σηlogτS\" -> 0.000000000000   ,  \"σηlogτN\" -> 0.000000000000   ,  \"σlogτ1\" -> 0.000000000000   ,  \"σlogτS\" -> 0.000000000000   ,  \"σlogτN\" -> 0.000000000000   ,  \"σητ1\" -> 0.000000000000   ,  \"σητS \" -> 0.000000000000   ,  \"σητN\" -> 0.000000000000    |>   , \r\"IDS0379_210909_RAW_cal__ref_\" ->   <|    \"ζ\" -> 0.425625100321   ,  \"τ1\" -> 0.068543660714   ,  \"τS\" -> 0.058744737584   ,  \"τN\" -> 0.070392227244   ,  \"τC\" -> 0.000760428296   ,  \"κ0\" -> 0.000000000614   ,  \"mm1\" -> 0.000225582014   ,  \"mm2\" -> 0.025358510497   ,  \"mm3\" -> 0.227820894937   ,  \"T\" -> 0.148000000000   ,  \"B\" -> 8.000000000000   ,  \"θ\" -> 0.000000000000   ,  \"Reoff\" -> -114874585.635359108000   ,  \"Imoff\" -> 0.000000000000   ,  \"στ1\" -> 0.000034854333   ,  \"στS\" -> 0.000021687796   ,  \"στN\" -> 0.000018077177   ,  \"τ11 \" -> 0.000000000000   ,  \"τ12\" -> 0.000000000000   ,  \"τ22\" -> 0.000000000000   ,  \"τN1\" -> 0.000000000000   ,  \"τN2\" -> 0.000000000000   ,  \"σηlogτ1 \" -> 0.000000000000   ,  \"σηlogτS\" -> 0.000000000000   ,  \"σηlogτN\" -> 0.000000000000   ,  \"σlogτ1\" -> 0.000000000000   ,  \"σlogτS\" -> 0.000000000000   ,  \"σlogτN\" -> 0.000000000000   ,  \"σητ1\" -> 0.000000000000   ,  \"σητS \" -> 0.000000000000   ,  \"σητN\" -> 0.000000000000    |>   , \r\"IDS0379_210909_RAW_cal__sam_\" ->   <|    \"ζ\" -> 0.225699737863   ,  \"τ1\" -> 0.105340283181   ,  \"τS\" -> 0.080581728797   ,  \"τN\" -> 0.103261234048   ,  \"τC\" -> 0.001367459466   ,  \"κ0\" -> 0.000000000745   ,  \"mm1\" -> 0.000248975261   ,  \"mm2\" -> 0.035515573270   ,  \"mm3\" -> 0.296279465482   ,  \"T\" -> 0.148000000000   ,  \"B\" -> 8.000000000000   ,  \"θ\" -> 0.000000000000   ,  \"Reoff\" -> -47870481.927710846100   ,  \"Imoff\" -> 0.000000000000   ,  \"στ1\" -> 0.000000000000   ,  \"στS\" -> 0.000000000000   ,  \"στN\" -> 0.000000000000   ,  \"τ11 \" -> 0.000000000000   ,  \"τ12\" -> 0.000000000000   ,  \"τ22\" -> 0.000000000000   ,  \"τN1\" -> 0.000000000000   ,  \"τN2\" -> 0.000000000000   ,  \"σηlogτ1 \" -> 0.000000000000   ,  \"σηlogτS\" -> 0.000000000000   ,  \"σηlogτN\" -> 0.000000000000   ,  \"σlogτ1\" -> 0.000000000000   ,  \"σlogτS\" -> 0.000000000000   ,  \"σlogτN\" -> 0.000000000000   ,  \"σητ1\" -> 0.000000000000   ,  \"σητS \" -> 0.000000000000   ,  \"σητN\" -> 0.000000000000    |>   , \r\"IDS0380_210909_RAW_cal__ref_\" ->   <|    \"ζ\" -> 0.296352280059   ,  \"τ1\" -> 0.061572423860   ,  \"τS\" -> 0.035048599519   ,  \"τN\" -> 0.042254612748   ,  \"τC\" -> 0.000902434218   ,  \"κ0\" -> 0.000000000747   ,  \"mm1\" -> 0.000203161456   ,  \"mm2\" -> 0.019927495587   ,  \"mm3\" -> 0.142556396514   ,  \"T\" -> 0.168000000000   ,  \"B\" -> 8.000000000000   ,  \"θ\" -> 0.000000000000   ,  \"Reoff\" -> -60285714.285714268700   ,  \"Imoff\" -> 0.000000000000   ,  \"στ1\" -> 0.000032565063   ,  \"στS\" -> 0.000015719503   ,  \"στN\" -> 0.000016419375   ,  \"τ11 \" -> 0.000000000000   ,  \"τ12\" -> 0.000000000000   ,  \"τ22\" -> 0.000000000000   ,  \"τN1\" -> 0.000000000000   ,  \"τN2\" -> 0.000000000000   ,  \"σηlogτ1 \" -> 0.000000000000   ,  \"σηlogτS\" -> 0.000000000000   ,  \"σηlogτN\" -> 0.000000000000   ,  \"σlogτ1\" -> 0.000000000000   ,  \"σlogτS\" -> 0.000000000000   ,  \"σlogτN\" -> 0.000000000000   ,  \"σητ1\" -> 0.000000000000   ,  \"σητS \" -> 0.000000000000   ,  \"σητN\" -> 0.000000000000    |>   , \r\"IDS0380_210909_RAW_cal__sam_\" ->   <|    \"ζ\" -> 0.175751625392   ,  \"τ1\" -> 0.093635045165   ,  \"τS\" -> 0.061160146348   ,  \"τN\" -> 0.068664853746   ,  \"τC\" -> 0.001317909381   ,  \"κ0\" -> 0.000000000855   ,  \"mm1\" -> 0.000193962663   ,  \"mm2\" -> 0.031705338902   ,  \"mm3\" -> 0.215695607858   ,  \"T\" -> 0.168000000000   ,  \"B\" -> 8.000000000000   ,  \"θ\" -> 0.000000000000   ,  \"Reoff\" -> -37527108.433734938500   ,  \"Imoff\" -> 0.000000000000   ,  \"στ1\" -> 0.000000000000   ,  \"στS\" -> 0.000000000000   ,  \"στN\" -> 0.000000000000   ,  \"τ11 \" -> 0.000000000000   ,  \"τ12\" -> 0.000000000000   ,  \"τ22\" -> 0.000000000000   ,  \"τN1\" -> 0.000000000000   ,  \"τN2\" -> 0.000000000000   ,  \"σηlogτ1 \" -> 0.000000000000   ,  \"σηlogτS\" -> 0.000000000000   ,  \"σηlogτN\" -> 0.000000000000   ,  \"σlogτ1\" -> 0.000000000000   ,  \"σlogτS\" -> 0.000000000000   ,  \"σlogτN\" -> 0.000000000000   ,  \"σητ1\" -> 0.000000000000   ,  \"σητS \" -> 0.000000000000   ,  \"σητN\" -> 0.000000000000    |>   , \r\"IDS0381_210909_RAW_cal__ref_\" ->   <|    \"ζ\" -> 0.135442001180   ,  \"τ1\" -> 0.054536829593   ,  \"τS\" -> 0.027242617167   ,  \"τN\" -> 0.009575045282   ,  \"τC\" -> 0.001074749120   ,  \"κ0\" -> 0.000000001354   ,  \"mm1\" -> 0.000124377738   ,  \"mm2\" -> 0.023594165009   ,  \"mm3\" -> 0.073697356296   ,  \"T\" -> 0.250000000000   ,  \"B\" -> 8.000000000000   ,  \"θ\" -> 0.000000000000   ,  \"Reoff\" -> -15819277.108433738400   ,  \"Imoff\" -> 0.000000000000   ,  \"στ1\" -> 0.000111598282   ,  \"στS\" -> 0.000013161229   ,  \"στN\" -> 0.000059063513   ,  \"τ11 \" -> 0.000000000000   ,  \"τ12\" -> 0.000000000000   ,  \"τ22\" -> 0.000000000000   ,  \"τN1\" -> 0.000000000000   ,  \"τN2\" -> 0.000000000000   ,  \"σηlogτ1 \" -> 0.000000000000   ,  \"σηlogτS\" -> 0.000000000000   ,  \"σηlogτN\" -> 0.000000000000   ,  \"σlogτ1\" -> 0.000000000000   ,  \"σlogτS\" -> 0.000000000000   ,  \"σlogτN\" -> 0.000000000000   ,  \"σητ1\" -> 0.000000000000   ,  \"σητS \" -> 0.000000000000   ,  \"σητN\" -> 0.000000000000    |>   , \r\"IDS0381_210909_RAW_cal__sam_\" ->   <|    \"ζ\" -> 0.077362618852   ,  \"τ1\" -> 0.058638638627   ,  \"τS\" -> 0.035602410157   ,  \"τN\" -> 0.012932252536   ,  \"τC\" -> 0.001722606032   ,  \"κ0\" -> 0.000000001497   ,  \"mm1\" -> 0.000118727642   ,  \"mm2\" -> 0.027585733079   ,  \"mm3\" -> 0.084946215242   ,  \"T\" -> 0.250000000000   ,  \"B\" -> 8.000000000000   ,  \"θ\" -> 0.000000000000   ,  \"Reoff\" -> -9843373.493975907570   ,  \"Imoff\" -> 0.000000000000   ,  \"στ1\" -> 0.000000000000   ,  \"στS\" -> 0.000000000000   ,  \"στN\" -> 0.000000000000   ,  \"τ11 \" -> 0.000000000000   ,  \"τ12\" -> 0.000000000000   ,  \"τ22\" -> 0.000000000000   ,  \"τN1\" -> 0.000000000000   ,  \"τN2\" -> 0.000000000000   ,  \"σηlogτ1 \" -> 0.000000000000   ,  \"σηlogτS\" -> 0.000000000000   ,  \"σηlogτN\" -> 0.000000000000   ,  \"σlogτ1\" -> 0.000000000000   ,  \"σlogτS\" -> 0.000000000000   ,  \"σlogτN\" -> 0.000000000000   ,  \"σητ1\" -> 0.000000000000   ,  \"σητS \" -> 0.000000000000   ,  \"σητN\" -> 0.000000000000    |>   , \r\"IDS0382_210909_RAW_cal__ref_\" ->   <|    \"ζ\" -> 0.083327700805   ,  \"τ1\" -> 0.049870021008   ,  \"τS\" -> 0.024726462582   ,  \"τN\" -> 0.005137571358   ,  \"τC\" -> 0.001213133652   ,  \"κ0\" -> 0.000000001736   ,  \"mm1\" -> 0.000089554374   ,  \"mm2\" -> 0.023106179536   ,  \"mm3\" -> 0.060239955976   ,  \"T\" -> 0.300000000000   ,  \"B\" -> 8.000000000000   ,  \"θ\" -> 0.000000000000   ,  \"Reoff\" -> -7659638.554216861730   ,  \"Imoff\" -> 0.000000000000   ,  \"στ1\" -> 0.000221537334   ,  \"στS\" -> 0.000014924990   ,  \"στN\" -> 0.000118586370   ,  \"τ11 \" -> 0.000000000000   ,  \"τ12\" -> 0.000000000000   ,  \"τ22\" -> 0.000000000000   ,  \"τN1\" -> 0.000000000000   ,  \"τN2\" -> 0.000000000000   ,  \"σηlogτ1 \" -> 0.000000000000   ,  \"σηlogτS\" -> 0.000000000000   ,  \"σηlogτN\" -> 0.000000000000   ,  \"σlogτ1\" -> 0.000000000000   ,  \"σlogτS\" -> 0.000000000000   ,  \"σlogτN\" -> 0.000000000000   ,  \"σητ1\" -> 0.000000000000   ,  \"σητS \" -> 0.000000000000   ,  \"σητN\" -> 0.000000000000    |>   , \r\"IDS0382_210909_RAW_cal__sam_\" ->   <|    \"ζ\" -> 0.054029770351   ,  \"τ1\" -> 0.051440847518   ,  \"τS\" -> 0.032079834642   ,  \"τN\" -> 0.007150632998   ,  \"τC\" -> 0.002202148776   ,  \"κ0\" -> 0.000000001884   ,  \"mm1\" -> 0.000106291219   ,  \"mm2\" -> 0.027352636275   ,  \"mm3\" -> 0.067534149597   ,  \"T\" -> 0.300000000000   ,  \"B\" -> 8.000000000000   ,  \"θ\" -> 0.000000000000   ,  \"Reoff\" -> 0.000000000000   ,  \"Imoff\" -> 0.000000000000   ,  \"στ1\" -> 0.000000000000   ,  \"στS\" -> 0.000000000000   ,  \"στN\" -> 0.000000000000   ,  \"τ11 \" -> 0.000000000000   ,  \"τ12\" -> 0.000000000000   ,  \"τ22\" -> 0.000000000000   ,  \"τN1\" -> 0.000000000000   ,  \"τN2\" -> 0.000000000000   ,  \"σηlogτ1 \" -> 0.000000000000   ,  \"σηlogτS\" -> 0.000000000000   ,  \"σηlogτN\" -> 0.000000000000   ,  \"σlogτ1\" -> 0.000000000000   ,  \"σlogτS\" -> 0.000000000000   ,  \"σlogτN\" -> 0.000000000000   ,  \"σητ1\" -> 0.000000000000   ,  \"σητS \" -> 0.000000000000   ,  \"σητN\" -> 0.000000000000    |>   , \r\"IDS0383_210910_RAW_cal__ref_\" ->   <|    \"ζ\" -> 0.062724752087   ,  \"τ1\" -> 0.048607141774   ,  \"τS\" -> 0.023827543799   ,  \"τN\" -> 0.003390848411   ,  \"τC\" -> 0.001761568500   ,  \"κ0\" -> 0.000000002107   ,  
